vi "Set Duty Cycle.vi"   [LabVIEW 2013, in "LVH-LINX.lvlib"]
doc: "Set the duty cycle of the specified PWM channel(s). \n\nA duty cycle of 0 coresponds to 0% on and a duty cycle of 255 coresponds to 100% on."
uses:
  <vilib>/LabVIEW Hacker/LINX/LVH-LINX.lvlib
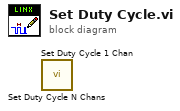
[diagram p0: block diagram]
diagram:
  n1 = call <vilib>:"Set Duty Cycle N Chans.vi"() -> ()  [unwired: 10 in, 2 out]
  n2 = call <vilib>:"Set Duty Cycle 1 Chan.vi"() -> ()  [unwired: 10 in, 2 out]
